vi "New.vi"(8 "error in (no error)":errorcluster, 11 "Termination Reason":T1={"Reason"=enum."Goodbye Received", "Reason URI"="wamp.error.protocol_violation", "Message"=""}) -> (0 "error out":errorcluster, 3 "Abort JSON out":refnum<class "Abort JSON.lvclass">)   [LabVIEW 2020, in "wamplv.lvlib" / "Abort JSON.lvclass"]
uses:
  Abort JSON.lvclass
  Abort JSON.lvclass/Abort JSON.ctl
  WAMP Client/Private/TypeDef/Termination Reason Enum.ctl
  WAMP Client/WAMP Client.lvclass
  WAMP Client/API/TypeDefs/Termination Reason.ctl
  wamplv.lvlib
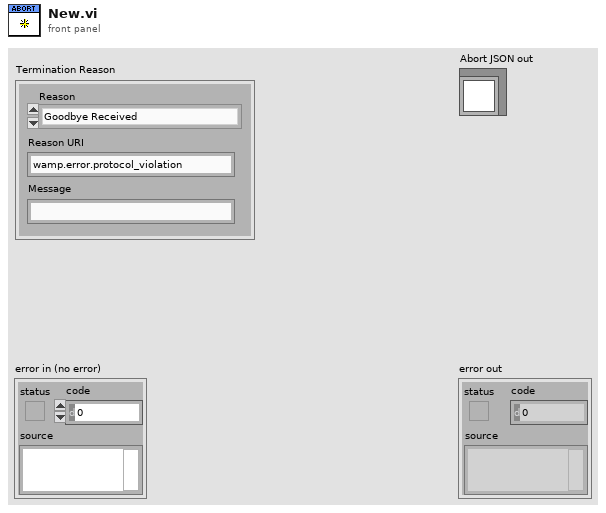
[diagram p1: front panel]
types:
  T1 = typedef "wamplv.lvlib/Termination Reason.ctl" = cluster{"Reason":T2, "Reason URI":string, "Message":string}
  T2 = typedef "wamplv.lvlib/WAMP Client.lvclass/Termination Reason Enum.ctl" = enum16{"Goodbye Received", "Abort Received", "Send Goodbye", "Send Abort", "Read Loop Failure", "Write Loop Failure", "Message Loop Failure", "wamplv aborted"}
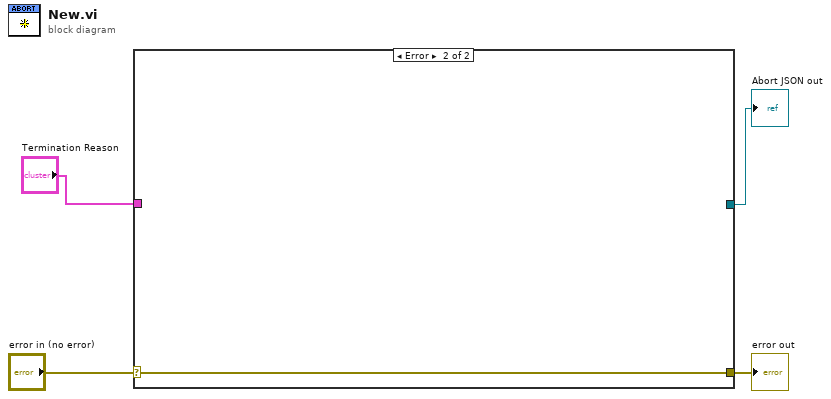
[diagram p0: block diagram]
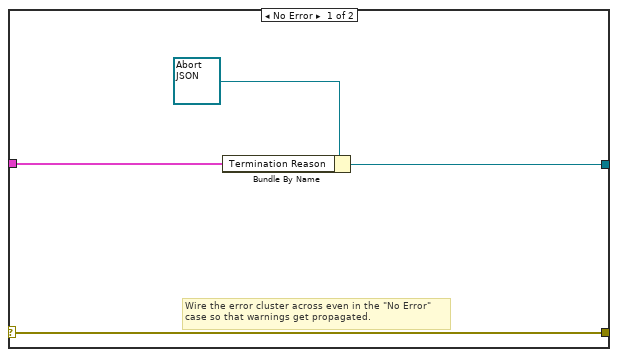
[diagram p2: hidden frame]
diagram:
  n1 = case shown="Error" "error in (no error)" {
    selector: "error in (no error)" -> [w8 w9]
    tunnel: [w8 w9] -> w3
    tunnel: "Termination Reason" -> [w6 _]
    tunnel: [w5 _] -> w1
    frame No Error {
      # "Wire the error cluster across even in the \"No Error\"\ncase so that warnings get propagated."
      n2 = Bundle By Name(cluster=refnum<class "Abort JSON.lvclass"> refnum ("wamplv.lvlib:Abort JSON.lvclass"), "Termination Reason"=w6) -> (w5:refnum<class "Abort JSON.lvclass">)
    }
    frame Error {
    }
  }
  "error out" <- w3
  "Abort JSON out" <- w1
